vi "PXDAC4800_BeginRamPlaybackXD48.vi"(2 "Playback bytes":u32, 3 "ram length bytes":u32, 4 "ram offset bytes":u32, 5 "Handle":i32) -> (0 "Status":i32, 1 "Handle Out":u32)   [LabVIEW 2016]
uses:
  PXDAC4800.dll
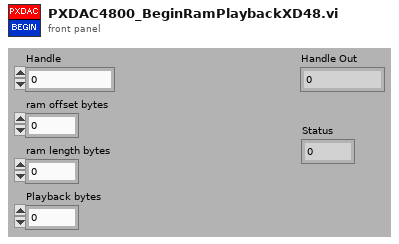
[diagram p1: front panel]
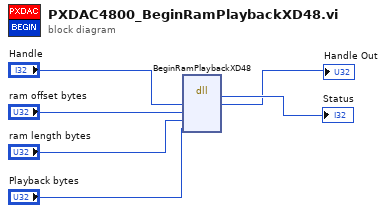
[diagram p0: block diagram]
diagram:
  n1 = dll-call lib="PXDAC4800.dll" fn="BeginRamPlaybackXD48"("Handle"="Handle", "ram_offset_bytes"="ram offset bytes", "ram_length_bytes"="ram length bytes", "playback_bytes"="Playback bytes") -> (→"Status":i32, "Handle"=→"Handle Out":u32)  [unwired: 6 in, 2 out]
